vi "UI Panels - Set Splitter Position.vi"(7 "index":i32, 8 "error in (no error)":errorcluster, 10 "Splitter Position":i32, 11 "Panels_XControl":refnum<vi>) -> (0 "error out":errorcluster, 3 "Panels_XControl":refnum<vi>)   [LabVIEW 2009, in "UI Panels.lvlib"]
uses:
  UI Panels.lvlib
  Panels_XControl.xctl
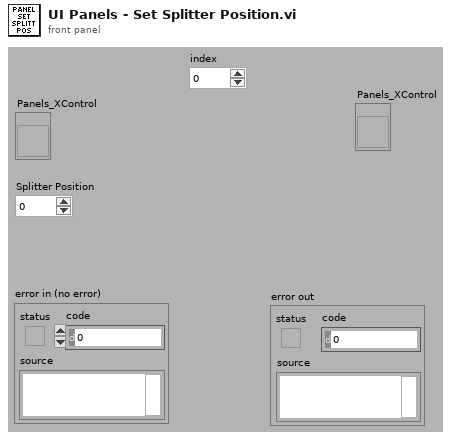
[diagram p1: front panel]
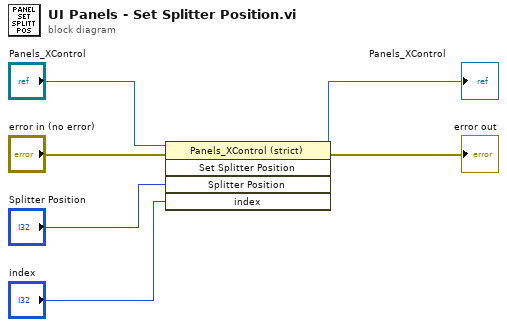
[diagram p0: block diagram]
diagram:
  n1 = invoke on="Invoke Node" class="Panels_XControl (strict)" method="Set Splitter Position"(reference="Panels_XControl", error in="error in (no error)", "Splitter Position"="Splitter Position", "index"="index") -> (reference out=→"Panels_XControl":refnum<vi>, error out=→"error out":errorcluster)  [unwired: 1 in, 3 out]
